vi "Center Calculated Distance.vi"(10 "Camera Distance\nfrom Ground (in)":dbl, 11 "Normalized Rect":T1) -> (2 "Distance (ft)":dbl, 3 "Distance Right (ft)":dbl)   [LabVIEW 2015]
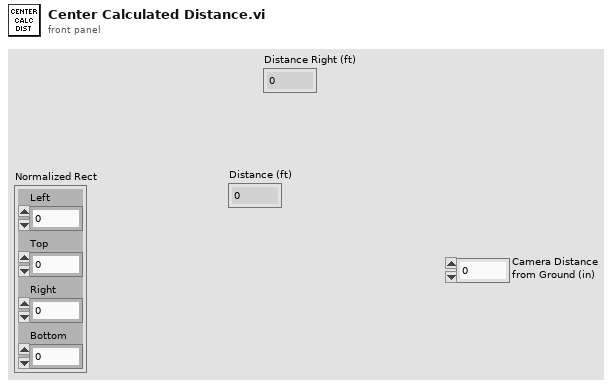
[diagram p1: front panel]
types:
  T1 = cluster{"Left":dbl, "Top":dbl, "Right":dbl, "Bottom":dbl}
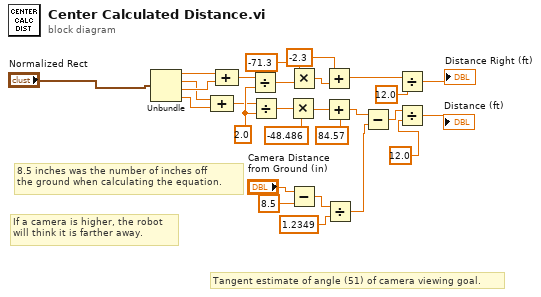
[diagram p0: block diagram]
diagram:
  w24 = 2.0
  # "If a camera is higher, the robot \nwill think it is farther away."
  # "8.5 inches was the number of inches off \nthe ground when calculating the equation."
  # "Tangent estimate of angle (51) of camera viewing goal."
  n1 = Unbundle("Normalized Rect") -> ("Left"=w28:dbl, "Top"=w25:dbl, "Right"=w27:dbl, "Bottom"=w26:dbl)
  n2 = Compound Arithmetic op=ADD(w25, w26) -> (w22:dbl)
  n3 = Compound Arithmetic op=ADD(w28, w27) -> (w23:dbl)
  n4 = Divide(x=w23, y=w24) -> (x/y=w16:dbl)
  n5 = Divide(x=w22, y=w24) -> (x/y=w20:dbl)
  n6 = Multiply(x=w20, y=-48.486) -> (x*y=w18:dbl)
  n7 = Multiply(x=-71.3, y=w16) -> (x*y=w15:dbl)
  n8 = Subtract(x="Camera Distance\nfrom Ground (in)", y=8.5) -> (x-y=w4:dbl)
  n9 = Add(x=-2.3, y=w15) -> (x+y=w12:dbl)
  n10 = Add(x=w18, y=84.57) -> (x+y=w7:dbl)
  n11 = Divide(x=w4, y=1.2349) -> (x/y=w2:dbl)
  n12 = Subtract(x=w7, y=w2) -> (x-y=w1:dbl)
  n13 = Divide(x=w12, y=12.0) -> (x/y=→"Distance Right (ft)":dbl)
  n14 = Divide(x=w1, y=12.0) -> (x/y=→"Distance (ft)":dbl)
